vi "Check_Channel.vi"(1 "Channels enabled":cluster{"A enabled":bool, "B enabled":bool}, 2 "Requested Channel":dbl) -> (0 "Boolean":bool)   [LabVIEW 2011]
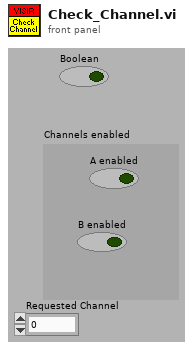
[diagram p1: front panel]
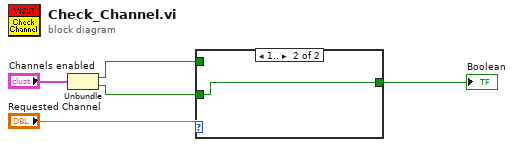
[diagram p0: block diagram]
diagram:
  n1 = Unbundle("Channels enabled") -> ("A enabled"=w2:bool, "B enabled"=w1:bool)
  n2 = case shown="1.." "Requested Channel" {
    tunnel: w1 -> [_ w7]
    tunnel: w2 -> [w6 _]
    tunnel: [w6 w7] -> w5
    frame ..0 {
    }
    frame 1.. {
    }
  }
  "Boolean" <- w5
